vi "Close Data File.vi"(8 "error in":errorcluster, 11 "File Refnum In":refnum<file>) -> (0 "error out":errorcluster)   [LabVIEW 2018]
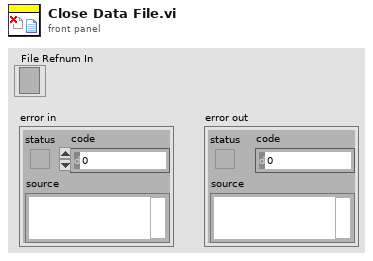
[diagram p1: front panel]
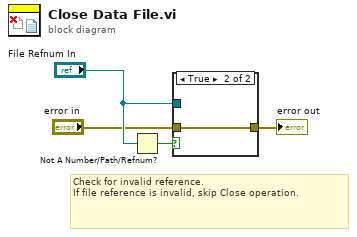
[diagram p0: block diagram]
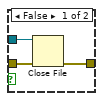
[diagram p2: hidden frame]
diagram:
  # "Check for invalid reference. \nIf file reference is invalid, skip Close operation."
  n1 = Not A Number/Path/Refnum?(number/path/refnum="File Refnum In") -> (NaN/Path/Refnum?=w4:bool)
  n2 = case shown="True" w4 {
    tunnel: "error in" -> [w7 w8]
    tunnel: "File Refnum In" -> [w6 _]
    tunnel: [w5 w8] -> w2
    frame False {
      n3 = Close File(refnum=w6, error in=w7) -> (error out=w5:errorcluster)  [unwired: 1 out]
    }
    frame True {
    }
  }
  "error out" <- w2
